vi "Name.vi"(8 "error in (no error)":errorcluster, 11 "Formatting Handler in":refnum<class "Formatting Handler.lvclass">) -> (0 "error out":errorcluster, 2 "class name":string, 3 "Formatting Handler out":refnum<class "Formatting Handler.lvclass">)   [LabVIEW 2018, in "GLog.lvlib" / "Formatting Handler.lvclass"]
uses:
  Formatting Handler.lvclass
  <vilib>/regexp/Match Regular Expression.xnode
panel:
  # "Connector Pane"
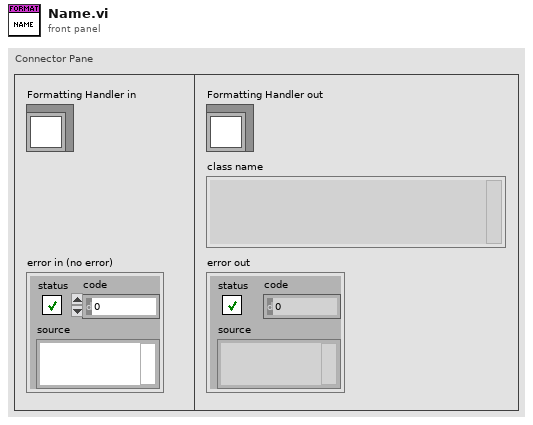
[diagram p1: front panel]
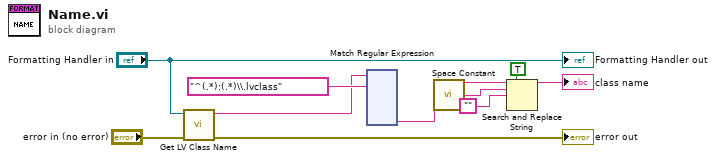
[diagram p0: block diagram]
diagram:
  n1 = call <vilib>:"Get LV Class Name.vi"("error in (no error)"="error in (no error)", "object"="Formatting Handler in") -> ("error out"=→"error out":errorcluster, "class name"=w6:string)  [unwired: 8 in]
  n2 = xnode "Match Regular Expression"("input string"=w6, "regular expression"="^(.*):(.*)\\.lvclass") -> ("submatch 2"=w2:string)  [unwired: 4 in, 6 out]
  n3 = call <vilib>:"Space Constant.vi"() -> ("String"=w5:string)
  n4 = Search and Replace String(replace all?=TRUE ("replace all? (F)"), input string=w2, search string=w5, replace string="") -> (result string=→"class name":string)  [unwired: 4 in, 3 out]
  "Formatting Handler out" <- "Formatting Handler in"
